vi "Write Voltage.vi"(8 "error in (no error)":errorcluster, 10 "Voltage":dbl[unit], 11 "Set Output Voltage Msg in":refnum<class "Set Output Voltage Msg.lvclass">) -> (0 "error out":errorcluster, 3 "Set Output Voltage Msg out":refnum<class "Set Output Voltage Msg.lvclass">)   [LabVIEW 2016, in "BNT_DAQmx.lvlib" / "Set Output Voltage Msg.lvclass"]
uses:
  Set Output Voltage Msg.lvclass
  Set Output Voltage Msg.lvclass/Set Output Voltage Msg.ctl
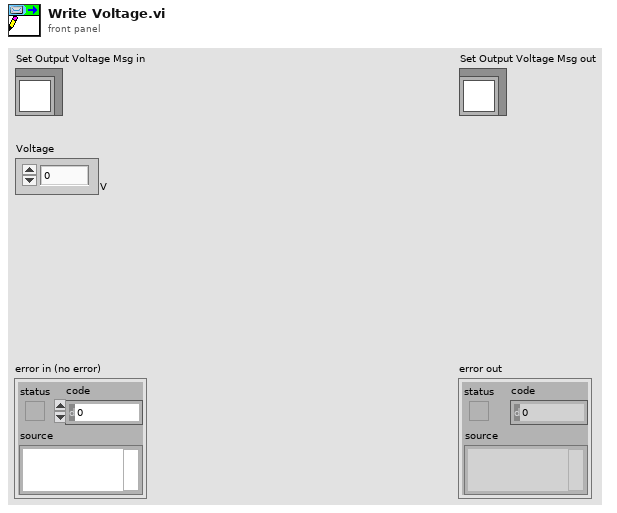
[diagram p1: front panel]
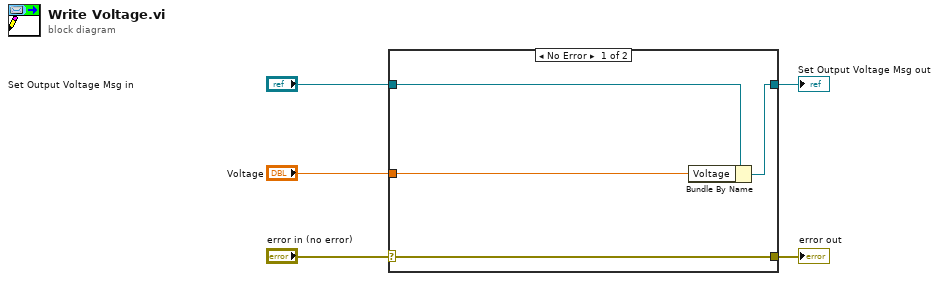
[diagram p0: block diagram]
diagram:
  n1 = case shown="No Error" "error in (no error)" {
    selector: "error in (no error)" -> [w9 w10]
    tunnel: [w9 w10] -> w4
    tunnel: [w7 w11] -> w2
    tunnel: "Set Output Voltage Msg in" -> [w8 w11]
    tunnel: "Voltage" -> [w6 _]
    frame No Error {
      n2 = Bundle By Name(cluster=w8, "Voltage"=w6) -> (w7:refnum<class "Set Output Voltage Msg.lvclass">)
    }
    frame Error {
    }
  }
  "error out" <- w4
  "Set Output Voltage Msg out" <- w2
